vi "Read Result.vi"(8 "error in (no error)":errorcluster, 11 "Process Object in":refnum<class "Process Object.lvclass">) -> (0 "error out":errorcluster, 2 "Acquired Result.lvclass":refnum<class "Acquired Result.lvclass">, 3 "Process Object out":refnum<class "Process Object.lvclass">)   [LabVIEW 2016, in "Process Object.lvclass"]
uses:
  Process Object.lvclass
  Results/Acquired Result/Acquired Result.lvclass
  Process Object.lvclass/Process Object.ctl
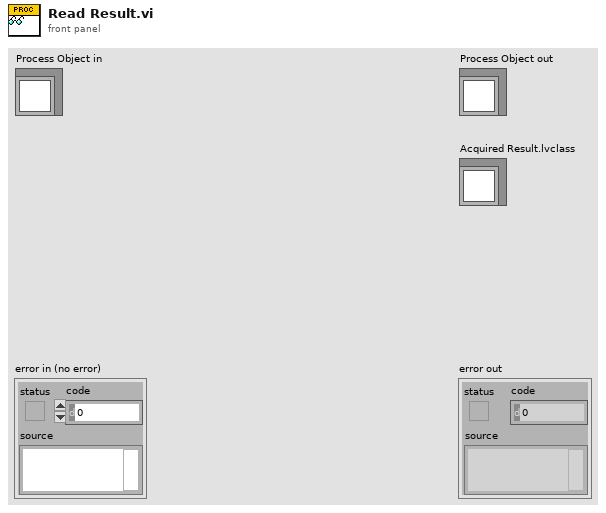
[diagram p1: front panel]
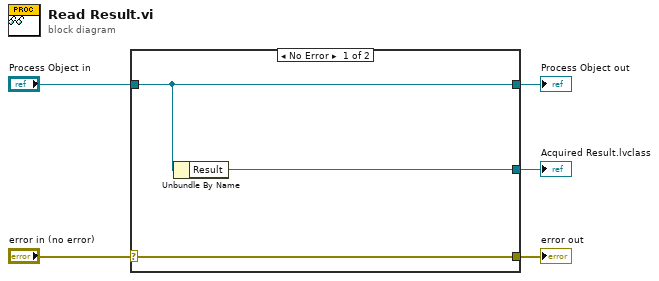
[diagram p0: block diagram]
diagram:
  n1 = case shown="No Error" "error in (no error)" {
    selector: "error in (no error)" -> [w8 w9]
    tunnel: [w8 w9] -> w4
    tunnel: [w7 w10] -> w2
    tunnel: "Process Object in" -> [w7 w10]
    tunnel: [w6 _] -> w1
    frame No Error {
      n2 = Unbundle By Name(w7) -> ("Result"=w6:refnum<class "Acquired Result.lvclass">)
    }
    frame Error {
    }
  }
  "error out" <- w4
  "Process Object out" <- w2
  "Acquired Result.lvclass" <- w1
